vi "Get_Setting_Power_dBm.vi"(8 "error in (no error)":errorcluster, 11 ".NET Reference in":refnum<k24>) -> (0 "error out":errorcluster, 2 "pow out":dbl, 3 "Reference out":refnum<k24>)   [LabVIEW 2017]
uses:
  C:/Users/Ssantec_Test/Documents/Instrument_DLL_Sample_Labview_20250826_Ver1.5.0_x64/DLL/InstrumentDLL.dll
  DLL/InstrumentDLL.dll
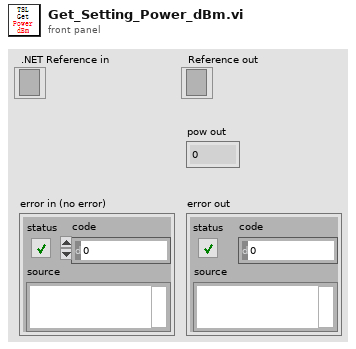
[diagram p1: front panel]
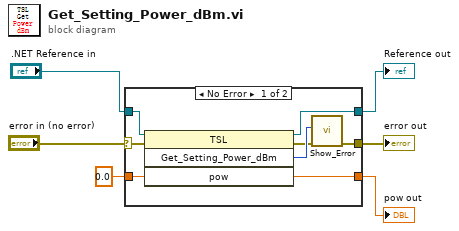
[diagram p0: block diagram]
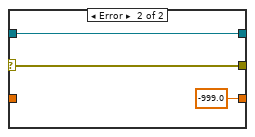
[diagram p2: hidden frame]
diagram:
  n1 = case shown="No Error" "error in (no error)" {
    selector: "error in (no error)" -> [w7 w17]
    tunnel: [w14 -999.0 ("pow")] -> w6
    tunnel: ".NET Reference in" -> [w13 w16]
    tunnel: [w12 w16] -> w4
    tunnel: [w8 w17] -> w3
    tunnel: 0.0 ("pow") -> [w11 _]
    frame No Error {
      n2 = invoke on="调用节点" class="TSL" method="Get_Setting_Power_dBm"(reference=w13, error in=w7, "pow"=w11) -> (reference out=w12:refnum<k24>, error out=w9:errorcluster, "Get_Setting_Power_dBm"=w10:i32, "pow"=w14:dbl)  [unwired: 1 in]
      n3 = call "Show_Error.vi"("error in (no error)"=w9, "Error"=w10) -> ("error out"=w8:errorcluster)  [unwired: 9 in]
    }
    frame Error {
    }
  }
  "pow out" <- w6
  "Reference out" <- w4
  "error out" <- w3
